vi "Test CameraTool Get Fiducial.vi"() -> ()   [LabVIEW 2011]
uses:
  Config Manager Class/Type Definitions/Fiducial Type.ctl
  CameraTool Class.lvclass
  Vec3d Class/Vec3d Class.lvclass
  Gantry Class/Gantry Class.lvclass
panel:
  out "Fiducial Position":cluster{"X":dbl, "Y":dbl, "Z":dbl}
  out "Routine Running":bool
  in  "Home First?":bool
  in  "Config Folder":path=path "C:/Users/Husker/Desktop/gantry/Config"
  out "error out":errorcluster
  out "Image Preview":T1(plugin-control)
  in  "Find Fiducial":bool
  in  "stop":bool
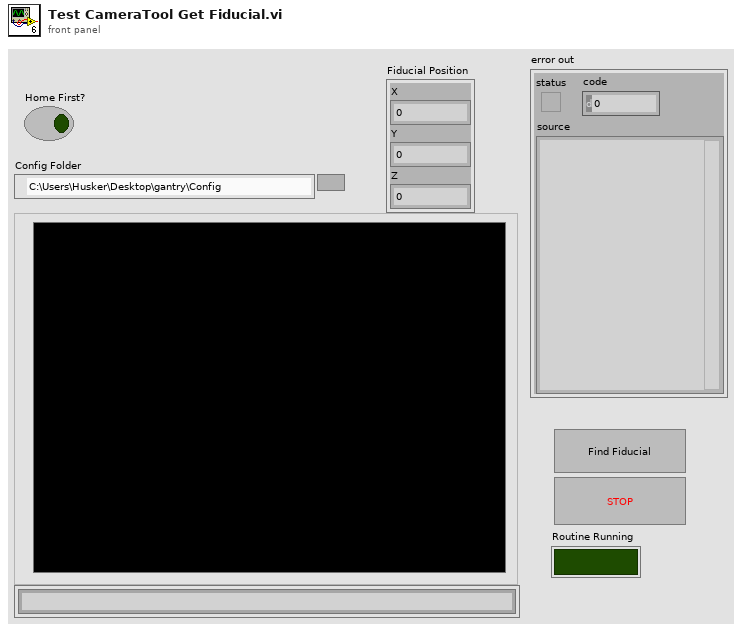
[diagram p1: front panel]
types:
  T1 = typedef "IMAQ Image.ctl" = refnum<image>
  T2 = typedef "Fiducial Type.ctl" = enum16{"HDI", "BBM"}
  T3 = typedef "Physical Image.ctl" = cluster{"Image Position":refnum<class "Vec3d Class.lvclass">, "Image Reference":T1, "Field of View":cluster{"x(mm)":dbl, "y(mm)":dbl}}
  T4 = typedef "Fiducial with Source.ctl" = cluster{"Fiducial Image Coordinate":refnum<class "Vec3d Class.lvclass">, "Fiducial Source":enum16{"Pattern Recognition", "User", "Error", "Default"}}
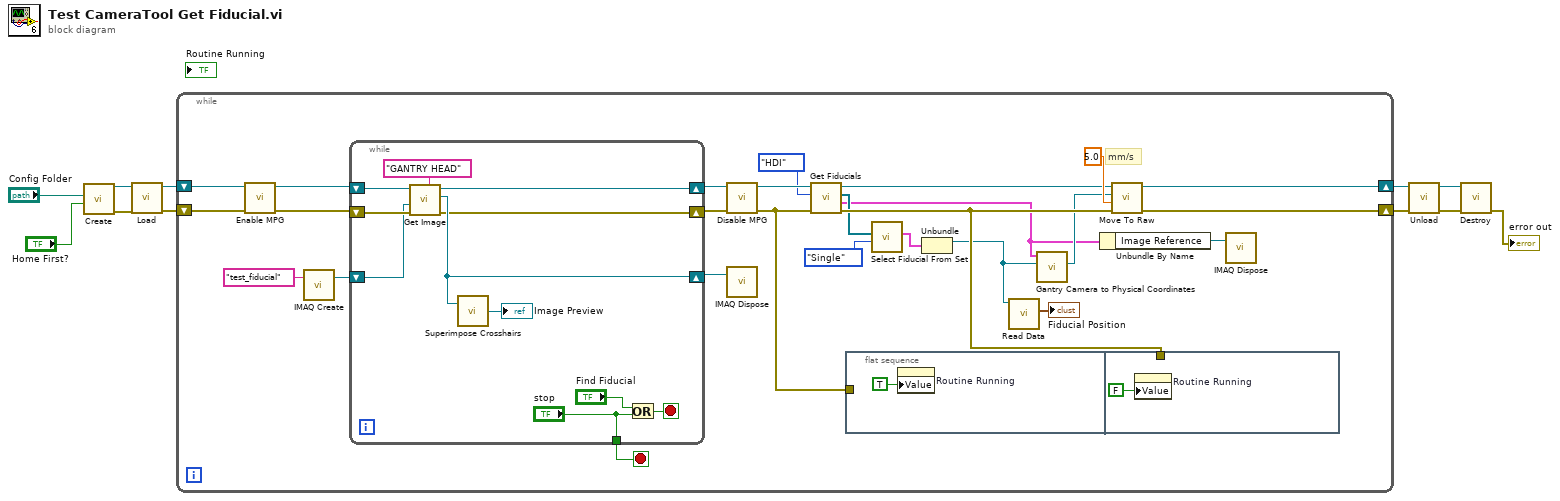
[diagram p0: block diagram]
diagram:
  n1 = call "Create.vi"("HOME?"="Home First?", "Config Folder"="Config Folder") -> ("error out"=w10:errorcluster, "Gantry out"=w11:refnum<class "Gantry Class.lvclass">)  [unwired: 8 in]
  n2 = call "Load.vi"("error in"=w10, "Gantry In"=w11) -> ("error out"=w8:errorcluster, "CameraTool out"=w9:refnum<class "CameraTool Class.lvclass">)  [unwired: 8 in]
  n3 = while {
    shift-right: [w19] -> w1
    shift-left: w9 -> [w34]
    shift-right: [w37] -> w7
    shift-left: w8 -> [w33]
    stop <- w22 stop-if-true
    # "mm/s"
    n4 = call-dynamic "Enable MPG.vi"("error in (no error)"=w33, "Gantry Class in"=w34) -> ("error out"=w31:errorcluster, "Gantry Class out"=w32:refnum<class "CameraTool Class.lvclass">)  [unwired: 8 in]
    n5 = call "IMAQ Create"("Image Name"="test_fiducial") -> ("New Image"=w24:T1)  [unwired: 4 in, 1 out]
    n6 = while {
      shift-right: [w48] -> w30
      shift-left: w32 -> [w50]
      shift-right: [w41] -> w28
      shift-left: w31 -> [w47]
      shift-right: [w43] -> w26
      shift-left: w24 -> [w44]
      tunnel: ["stop"] -> w22
      stop <- w45 stop-if-true
      n7 = call-dynamic "Get Image.vi"("error in"=w47, "Image In"=w44, "Camera Name"="GANTRY HEAD", "Gantry in"=w50) -> ("error out"=w41:errorcluster, "Image Out"=w43:T1, "Gantry out"=w48:refnum<class "CameraTool Class.lvclass">)  [unwired: 4 in, 1 out]
      n8 = call "Superimpose Crosshairs.vi"("Refnum in"=w43) -> ("Refnum out"=→"Image Preview":T1)  [unwired: 1 in]
      n9 = Or(x="Find Fiducial", y="stop") -> (x .or. y?=w45:bool)
    }
    n10 = call-dynamic "Disable MPG.vi"("error in"=w28, "Gantry in"=w30) -> ("error out"=w27:errorcluster, "Gantry out"=w29:refnum<class "CameraTool Class.lvclass">)  [unwired: 8 in]
    n11 = call "IMAQ Dispose"("Image"=w26) -> ()  [unwired: 5 in, 1 out]
    n12 = call "Get Fiducials.vi"("error in"=w27, "Fiducial Type"=Fiducial_Type."HDI", "CameraTool In"=w29) -> ("error out"=w35:errorcluster, "Fiducial Image"=w16:T3, "Fiducial Image Positions"=w21:refnum<class "Vec3d Class.lvclass">[], "CameraTool Out"=w17:refnum<class "CameraTool Class.lvclass">)  [unwired: 3 in]
    n13 = flat-sequence {
      tunnel: w27 -> [_]
      tunnel: w35 -> [_]
      frame #0 {
        n14 = property on="Routine Running" class="Bool (strict)"("Value"=TRUE ("Focus Routine Running")) -> ()  [unwired: 2 in, 2 out]
      }
      frame #1 {
        n15 = property on="Routine Running" class="Bool (strict)"("Value"=FALSE ("Focus Routine Running")) -> ()  [unwired: 2 in, 2 out]
      }
    }
    n16 = call "Select Fiducial From Set.vi"("Selection Criteria"=enum16{"Single", "Top", "Bottom"}."Single", "Fiducial Centers"=w21) -> ("Fiducial with Source"=w14:T4)  [unwired: 8 in, 1 out]
    n17 = Unbundle(w14) -> ("Fiducial Image Coordinate"=w13:refnum<class "Vec3d Class.lvclass">)  [unwired: 1 out]
    n18 = call-dynamic "Read Data.vi"("Vec3d Class in"=w13) -> ("Data"=→"Fiducial Position":cluster{"X":dbl, "Y":dbl, "Z":dbl})  [unwired: 8 in, 2 out]
    n19 = call "Gantry Camera to Physical Coordinates.vi"("Image Coordinate"=w13, "Physical Image"=w16) -> ("Global Coordinate"=w18:refnum<class "Vec3d Class.lvclass">)  [unwired: 7 in, 2 out]
    n20 = Unbundle By Name(w16) -> ("Image Reference"=w15:T1)
    n21 = call-dynamic "Move To Raw.vi"("error in"=w35, "Speed"=5.0, "Destination"=w18, "Gantry in"=w17) -> ("error out"=w37:errorcluster, "Gantry out"=w19:refnum<class "CameraTool Class.lvclass">)  [unwired: 6 in]
    n22 = call "IMAQ Dispose"("Image"=w15) -> ()  [unwired: 5 in, 1 out]
  }
  n23 = call "Unload.vi"("error in"=w7, "CameraTool in"=w1) -> ("error out"=w5:errorcluster, "Gantry out"=w6:refnum<class "Gantry Class.lvclass">)  [unwired: 8 in]
  n24 = call "Destroy.vi"("error in"=w5, "Gantry Class in"=w6) -> ("error out"=→"error out":errorcluster)  [unwired: 9 in]
